vi "RFID MFRC522 Example.vi"   [LabVIEW 2014]
uses:
  QwaveSys_Interface/QwaveSys_Interface.lvlib
  QwaveSys_ESP8266/QwaveSys_ESP8266.lvlib
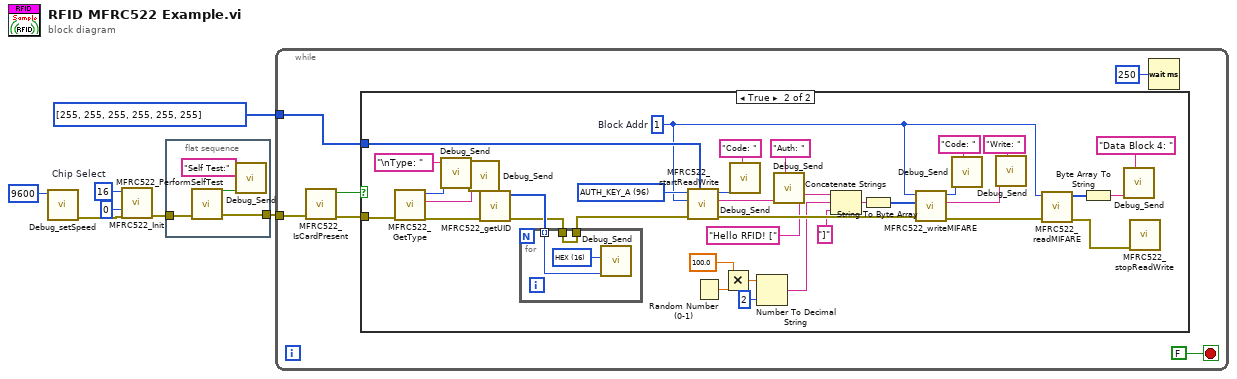
[diagram p0: block diagram]
diagram:
  w7 = u8 16  # Chip Select
  n1 = call "Debug_setSpeed.vi"("Speed"=u32 9600) -> ("error out"=w5:errorcluster)  [unwired: 10 in]
  n2 = call "MFRC522_Init.vi"("error in (no error)"=w5, "Reset"=u8 0, "Chip Select"=w7) -> ("error out"=w2:errorcluster)  [unwired: 8 in]
  n3 = flat-sequence {
    tunnel: w2 -> [w10]
    tunnel: [w9] -> w1
    frame #0 {
      n4 = call "MFRC522_PerformSelfTest.vi"("error in (no error)"=w10) -> ("error out"=w9:errorcluster, "status"=w8:bool)  [unwired: 9 in]
      n5 = call "Debug_Send.vi"("Name"="Self Test:", "DATA"=w8) -> ()  [unwired: 10 in]
    }
  }
  n6 = while {
    tunnel: w1 -> [w17]
    tunnel: u8[] [255, 255, 255, 255, 255, 255] ("Key (6 bytes)") -> [w12]
    stop <- FALSE stop-if-true
    n7 = call "MFRC522_IsCardPresent.vi"("error in (no error)"=w17) -> ("error out"=w16:errorcluster, "status"=w13:bool)  [unwired: 9 in]
    n8 = case shown="True" w13 {
      tunnel: w16 -> [_ w36]
      tunnel: w12 -> [_ w49]
      frame False {
      }
      frame True {
        w18 = u8 1  # Block Addr
        w51 = u16 96 items=["AUTH_KEY_A"=96, "AUTH_KEY_B"=97] ("Key")
        n9 = call "MFRC522_GetType.vi"("error in (no error)"=w36) -> ("error out"=w35:errorcluster, "Type Name"=w32:string, "Type"=w33:u8)  [unwired: 8 in]
        n10 = call "Debug_Send.vi"("Name"="\nType: ", "DATA"=w33) -> ()  [unwired: 10 in]
        n11 = call "Debug_Send.vi"("DATA"=w32) -> ()  [unwired: 11 in]
        n12 = call "MFRC522_getUID.vi"("error in (no error)"=w35) -> ("error out"=w20:errorcluster, "UID"=w34:u8[])  [unwired: 9 in]
        n13 = for {
          tunnel: w34 -> [w54] mode=indexing
          tunnel: w20 -> [w52]
          tunnel: [w52] -> w19
          w53 = u16 16 items=["DEC"=10, "HEX"=16, "OCT"=8, "BIN"=2] ("Option")
          n14 = call "Debug_Send.vi"("DATA"=w54, "Option"=w53) -> ()  [unwired: 10 in]
        }
        n15 = call "MFRC522_startReadWrite.vi"("Key (6 bytes)"=w49, "error in (no error)"=w19, "Block Address"=w18, "Key"=w51) -> ("error out"=w46:errorcluster, "Status Name"=w30:string, "Status Code"=w29:u8)  [unwired: 5 in]
        n16 = Random Number (0-1)() -> (number: 0 to 1=w44:dbl)
        n17 = Multiply(x=100.0, y=w44) -> (x*y=w42:dbl)
        n18 = call "Debug_Send.vi"("Name"="Code: ", "DATA"=w29) -> ()  [unwired: 10 in]
        n19 = Number To Decimal String(number=w42, width (-)=i16 2) -> (decimal integer string=w40:string)
        n20 = call "Debug_Send.vi"("Name"="Auth: ", "DATA"=w30) -> ()  [unwired: 10 in]
        n21 = Concatenate Strings("Hello RFID! [", w40, "]" ("string")) -> (w38:string)
        n22 = String To Byte Array(string=w38) -> (unsigned byte array=w45:u8[])
        n23 = call "MFRC522_writeMIFARE.vi"("error in (no error)"=w46, "Data (max 16 bytes)"=w45, "Block Address"=w18) -> ("error out"=w47:errorcluster, "Status Name"=w23:string, "Status Code"=w26:u8)  [unwired: 6 in]
        n24 = call "Debug_Send.vi"("Name"="Code: ", "DATA"=w26) -> ()  [unwired: 10 in]
        n25 = call "Debug_Send.vi"("Name"="Write: ", "DATA"=w23) -> ()  [unwired: 10 in]
        n26 = call "MFRC522_readMIFARE.vi"("error in (no error)"=w47, "Block Address"=w18) -> ("error out"=w50:errorcluster, "Data"=w48:u8[])  [unwired: 8 in]
        n27 = Byte Array To String(unsigned byte array=w48) -> (string=w22:string)
        n28 = call "Debug_Send.vi"("Name"="Data Block 4: ", "DATA"=w22) -> ()  [unwired: 10 in]
        n29 = call "MFRC522_stopReadWrite.vi"("error in (no error)"=w50) -> ()  [unwired: 10 in, 1 out]
      }
    }
    n30 = Wait (ms)(milliseconds to wait=u32 250) -> ()  [unwired: 1 out]
  }
